vi "TH_SaveVal.vi"(0 "Humidities In":dbl[](array[numeric]) format="%.2f", 1 "Temperatures In":dbl[](array[numeric]) format="%.2f", 2 "MeanTime (sec)":dbl format="%.2f") -> ()   [LabVIEW 2014]
uses:
  TH_Globals.vi
panel:
  out "Saving Data...":bool
  in  "Array Output":dbl[](array[numeric]) format="%.1f"
  out "StartTime":dbl format="%.2f"
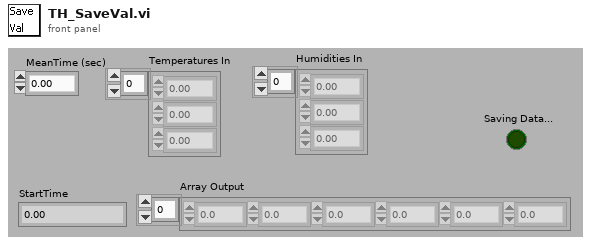
[diagram p1: front panel]
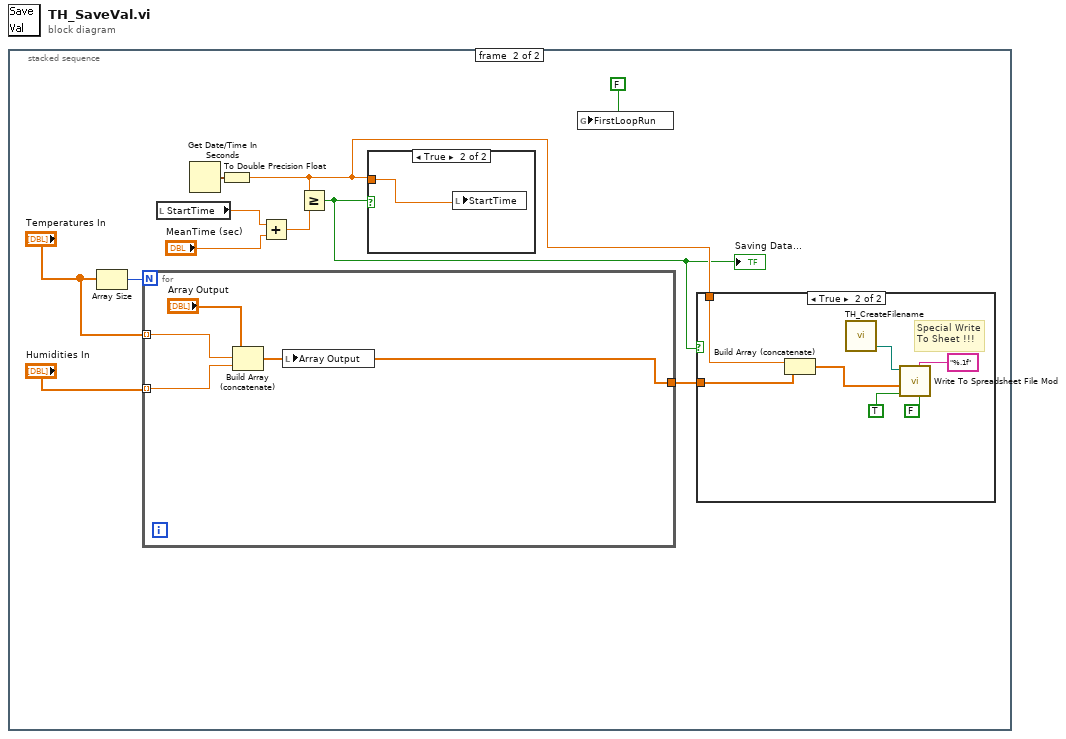
[diagram p0: block diagram]
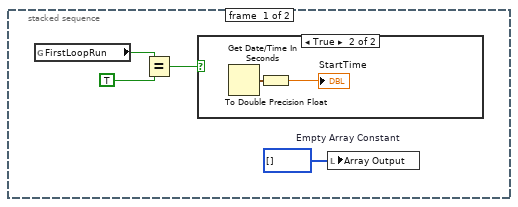
[diagram p2: hidden frame]
diagram:
  n1 = stacked-sequence {
    frame #0 {
      w1 = i32[] []  # Empty Array Constant
      n2 = global read "TH_Globals.vi" "FirstLoopRun"() -> (w4:bool)
      n3 = Equal?(x=w4, y=TRUE) -> (x = y?=w2:bool)
      n4 = case shown="True" w2 {
        frame False {
        }
        frame True {
          n5 = Get Date/Time In Seconds() -> (seconds since 1Jan1904=w5:timestamp)
          n6 = To Double Precision Float(number=w5) -> (double precision float=→"StartTime":dbl)
        }
      }
      n7 = local write "Array Output"(w1) -> ()
    }
    frame #1 {
      n8 = Array Size(array="Temperatures In") -> (size(s)=w17:i32)
      n9 = for {
        N: w17 -> [_]
        tunnel: "Temperatures In" -> [w28] mode=indexing
        tunnel: "Humidities In" -> [w27] mode=indexing
        tunnel: [w26] -> w10
        n10 = Build Array (concatenate)("Array Output", w28, w27) -> (w26:dbl[])
        n11 = local write "Array Output"(w26) -> ()
      }
      n12 = local read "StartTime"() -> (w13:dbl)
      n13 = Get Date/Time In Seconds() -> (seconds since 1Jan1904=w7:timestamp)
      n14 = To Double Precision Float(number=w7) -> (double precision float=w9:dbl)
      n15 = Add(x=w13, y="MeanTime (sec)") -> (x+y=w12:dbl)
      n16 = Greater Or Equal?(x=w9, y=w12) -> (x >= y?=w8:bool)
      "Saving Data..." <- w8
      n17 = case shown="True" w8 {
        tunnel: w9 -> [_ w25]
        frame False {
        }
        frame True {
          n18 = local write "StartTime"(w25) -> ()
        }
      }
      n19 = global write "TH_Globals.vi" "FirstLoopRun"(FALSE) -> ()
      n20 = case shown="True" w8 {
        tunnel: w10 -> [_ w20]
        tunnel: w9 -> [_ w19]
        frame False {
        }
        frame True {
          # "Special Write\nTo Sheet !!!"
          n21 = Build Array (concatenate)(w19, w20) -> (w24:dbl[])
          n22 = call "TH_CreateFilename.vi"() -> ("DataPath + Filename"=w18:path)  [unwired: 5 in, 2 out]
          n23 = call "Write To Spreadsheet File Mod.vi"("transpose? (no:F)"=FALSE, "format (%.3f)"="%.1f", "append to file? (new file:F)"=TRUE, "1D data"=w24, "file path (dialog if empty)"=w18) -> ()  [unwired: 3 in, 1 out]
        }
      }
    }
  }
